vi "Update Versions.vi"(7 "Versions":string[](array[string]), 8 "error in":errorcluster, 11 "Refnum in":refnum<k20>) -> (0 "error out":errorcluster, 3 "Refnum out":refnum<k20>)   [LabVIEW 2018, in "Serializer.lvclass"]
uses:
  Serializer.lvclass
  <vilib>/xml/Close Reference(Node).vi
  <vilib>/xml/NI_XML.lvlib
  <resource>/objmgr/DOMUserDefRef.rc
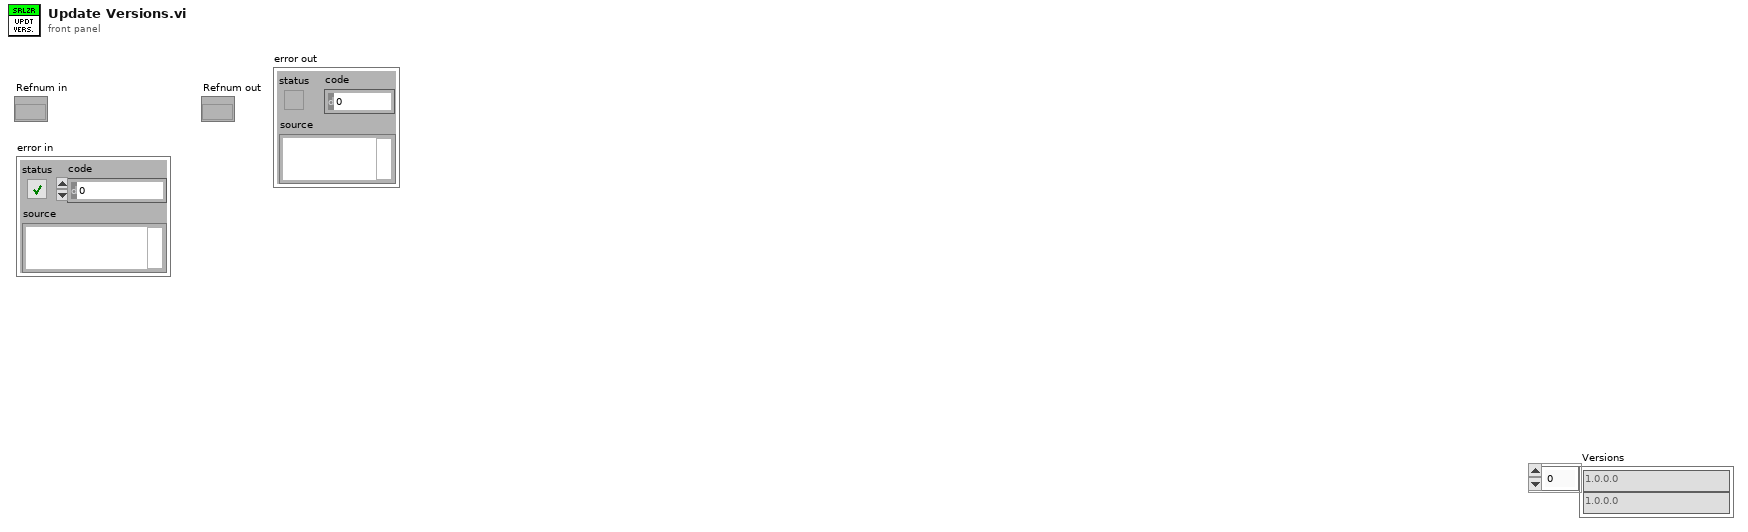
[diagram p1: front panel]
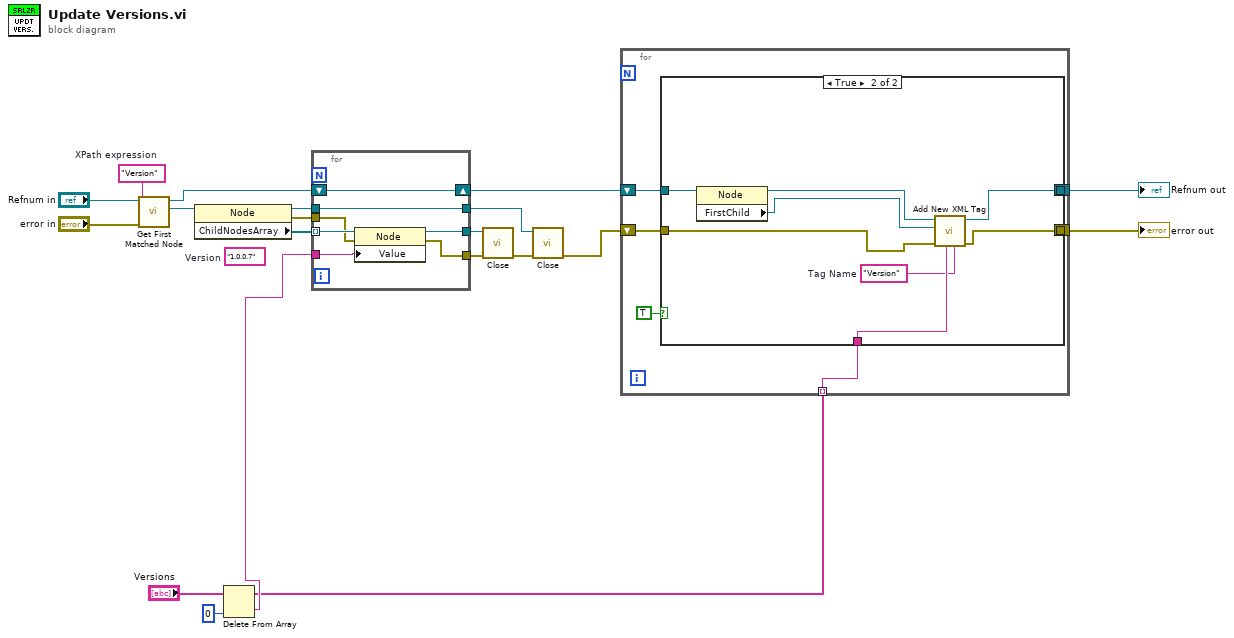
[diagram p0: block diagram]
diagram:
  (unwired) "1.0.0.7"  # Version
  w20 = "Version"  # XPath expression
  n1 = call <vilib>:"Get First Matched Node.vi"("error in (no error)"="error in", "XPath expression"=w20, "node in"="Refnum in") -> ("node result"=w6:refnum<k20>, "node out"=w19:refnum<k20>)  [unwired: 6 in, 1 out]
  n2 = property class="Node"(reference=w6) -> (reference out=w18:refnum<k20>, error out=w12:errorcluster, "ChildNodesArray"=w17:refnum<k20>[])  [unwired: 1 in]
  n3 = Delete From Array(array="Versions", index=0) -> (deleted portion=w3:string, array with subset deleted=w1:string[])  [unwired: 1 in]
  n4 = for {
    tunnel: w17 -> [w27] mode=indexing
    tunnel: w3 -> [w26]
    tunnel: w18 -> [w25]
    tunnel: [w25] -> w14
    shift-right: [w24] -> w10
    shift-left: w19 -> [w24]
    tunnel: [w23] -> w15
    tunnel: w12 -> [w22]
    tunnel: [w21] -> w11
    n5 = property class="Node"(reference=w27, error in=w22, "Value"=w26) -> (reference out=w23:refnum<k20>, error out=w21:errorcluster)
  }
  n6 = call-poly <vilib>:"Close.vi"("error in (no error)"=w11, "node"=w15) -> ("error out"=w13:errorcluster)  [unwired: 7 in]
  n7 = call-poly <vilib>:"Close.vi"("error in (no error)"=w13, "node"=w14) -> ("error out"=w8:errorcluster)  [unwired: 7 in]
  n8 = for {
    shift-right: [w29] -> w5
    shift-left: w10 -> [w33]
    shift-right: [w32] -> w9
    shift-left: w8 -> [w31]
    tunnel: w1 -> [w28] mode=indexing
    n9 = case shown="True" TRUE {
      tunnel: w33 -> [w35 w43]
      tunnel: [w35 w40] -> w29
      tunnel: w31 -> [w34 w38]
      tunnel: [w34 w39] -> w32
      tunnel: w28 -> [_ w37]
      frame False {
      }
      frame True {
        w36 = "Version"  # Tag Name
        n10 = property class="Node"(reference=w43) -> (reference out=w42:refnum<k20>, "FirstChild"=w41:refnum<k20>)  [unwired: 1 in, 1 out]
        n11 = call "Add New XML Tag.vi"("Tag Name"=w36, "Tag Data"=w37, "error in (no error)"=w38, "Owning Element"=w41, "DOM document"=w42) -> ("error out"=w39:errorcluster, "dup DOM document"=w40:refnum<k20>)  [unwired: 4 in, 1 out]
      }
    }
  }
  "Refnum out" <- w5
  "error out" <- w9
